vi "WaitPass.vi"(9 "balls":T1[](array[typedef])=[{"x"=-2165.869384765625, "y"=510.4085693359375, "timestamp"=timestamp(2082758857.4639893 s since 1904-01-01), "Vel_x"=0.0, "Vel_y"=0.0, "Pos Bola Est"=[]}], 10 "Target":dbl[](array[numeric]), 11 "Robot in":T2) -> (3 "Robot out":T2)   [LabVIEW 2016]
uses:
  Core/AI Robot.ctl
  Functions Enum.ctl
  AttackerStates.ctl
  Core/AI Ball.ctl
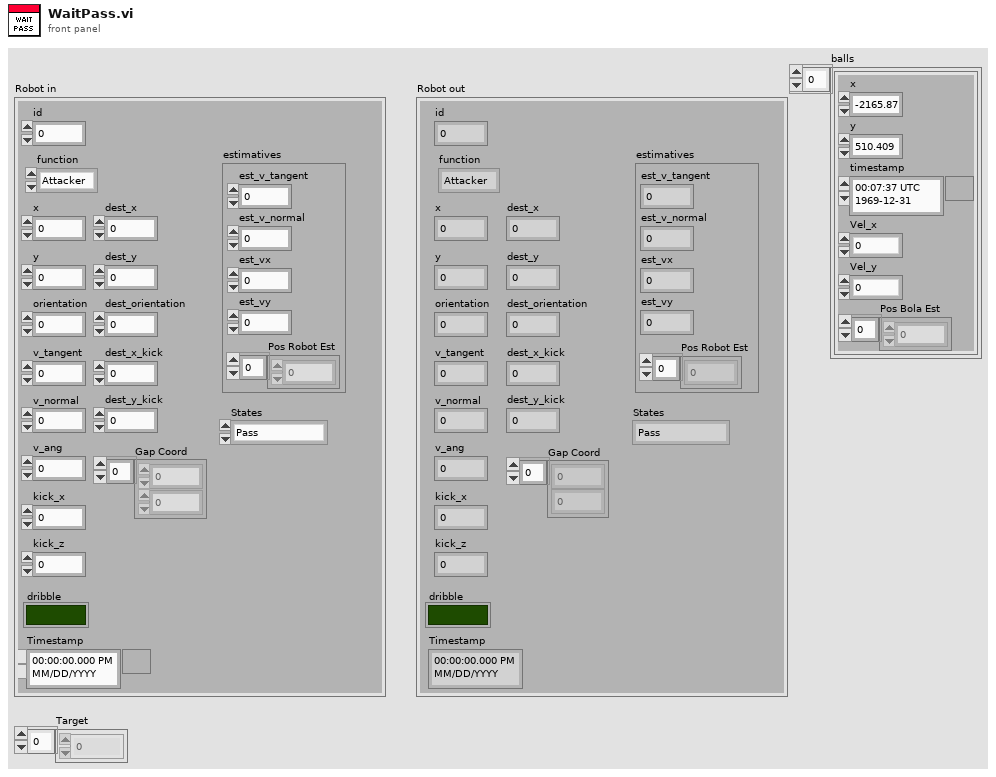
[diagram p1: front panel]
types:
  T1 = typedef "AI Ball.ctl" = cluster{"x":dbl, "y":dbl, "timestamp":timestamp, "Vel_x":dbl, "Vel_y":dbl, "Pos Bola Est":dbl[]}
  T2 = typedef "AI Robot.ctl" = cluster{"id":u32, "function":T3, "x":dbl, "y":dbl, "orientation":dbl, "v_tangent":dbl, "v_normal":dbl, "v_ang":dbl, "kick_x":dbl, "kick_z":dbl, "dribble":bool, "Timestamp":timestamp, "dest_x":dbl, "dest_y":dbl, "dest_orientation":dbl, "estimatives":cluster{"est_v_tangent":dbl, "est_v_normal":dbl, "est_vx":dbl, "est_vy":dbl, "Pos Robot Est":dbl[]}, "dest_x_kick":dbl, "dest_y_kick":dbl, "Gap Coord":dbl[], "States":T4}
  T3 = typedef "Functions Enum.ctl" = enum16{"Attacker", "Goalie", "Defender", "Striker", "Goto 0", "Dummy", "Kicker", "ZigZag"}
  T4 = typedef "AttackerStates.ctl" = enum16{"Pass", "GoToTangent", "BallGetting", "GoToKick", ""}
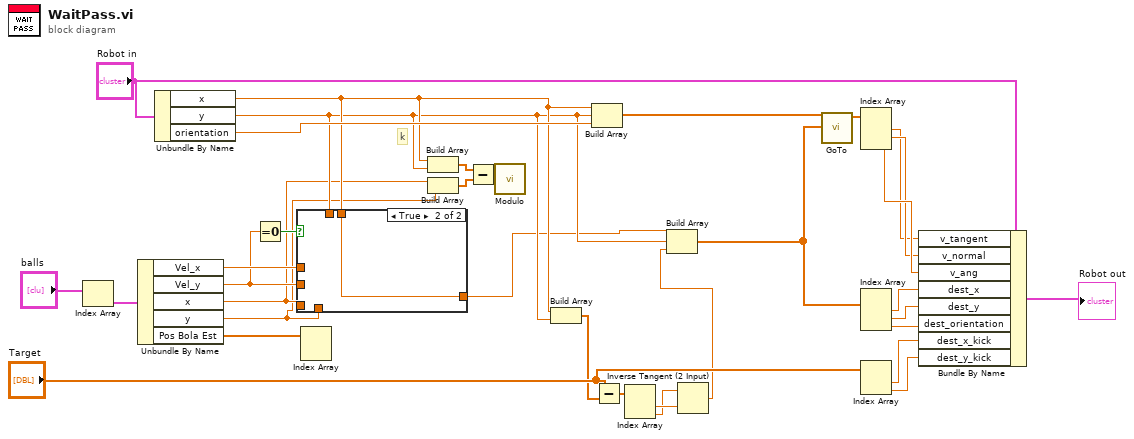
[diagram p0: block diagram]
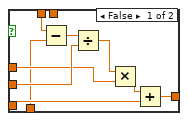
[diagram p2: hidden frame]
diagram:
  # "k"
  n1 = Index Array(array="balls") -> (element=w15:T1)  [unwired: 1 in]
  n2 = Unbundle By Name(w15) -> ("Vel_x"=w13:dbl, "Vel_y"=w9:dbl, "x"=w6:dbl, "y"=w5:dbl, "Pos Bola Est"=w14:dbl[])
  n3 = Unbundle By Name("Robot in") -> ("x"=w8:dbl, "y"=w7:dbl, "orientation"=w20:dbl)
  n4 = Equal To 0?(x=w9) -> (x = 0?=w10:bool)
  n5 = case shown="True" w10 {
    tunnel: w9 -> [w42 _]
    tunnel: w6 -> [w41 _]
    tunnel: w13 -> [w38 _]
    tunnel: [w37 w44] -> w1
    tunnel: w7 -> [w36 _]
    tunnel: w5 -> [w35 _]
    tunnel: w8 -> [_ w44]
    frame False {
      n6 = Subtract(x=w36, y=w35) -> (x-y=w43:dbl)
      n7 = Divide(x=w43, y=w42) -> (x/y=w39:dbl)
      n8 = Multiply(x=w39, y=w38) -> (x*y=w40:dbl)
      n9 = Add(x=w40, y=w41) -> (x+y=w37:dbl)
    }
    frame True {
    }
  }
  n10 = Index Array(array=w14) -> ()  [unwired: 2 in, 2 out]
  n11 = Build Array(w8, w7) -> (w4:dbl[])
  n12 = Build Array(w6, w5) -> (w3:dbl[])
  n13 = Subtract(x=w4, y=w3) -> (x-y=w2:dbl[])
  n14 = call "Modulo.vi"("2D vector"=w2) -> ()  [unwired: 10 in, 1 out]
  n15 = Build Array(w8, w7) -> (w19:dbl[])
  n16 = Build Array(w8, w7, w20) -> (w25:dbl[])
  n17 = Subtract(x="Target", y=w19) -> (x-y=w21:dbl[])
  n18 = Index Array(array=w21) -> (element #1=w23:dbl, element #2=w22:dbl)  [unwired: 2 in]
  n19 = Inverse Tangent (2 Input)(1:w23, 2:w22) -> (0:w12:dbl)
  n20 = Build Array(w1, w7, w12) -> (w11:dbl[])
  n21 = call "GoTo.vi"("Target"=w11, "Position"=w25) -> ("Output\nVelocity"=w24:dbl[])  [unwired: 8 in, 1 out]
  n22 = Index Array(array=w24) -> (element #1=w32:dbl, element #2=w33:dbl, element #3=w34:dbl)  [unwired: 3 in]
  n23 = Index Array(array=w11) -> (element #1=w29:dbl, element #2=w30:dbl, element #3=w31:dbl)  [unwired: 3 in]
  n24 = Index Array(array="Target") -> (element #1=w27:dbl, element #2=w28:dbl)  [unwired: 2 in]
  n25 = Bundle By Name(cluster="Robot in", "v_tangent"=w32, "v_normal"=w33, "v_ang"=w34, "dest_x"=w29, "dest_y"=w30, "dest_orientation"=w31, "dest_x_kick"=w27, "dest_y_kick"=w28) -> (→"Robot out":T2)
